vi "dos cmd test.vi"() -> ()   [LabVIEW 2010]
uses:
  <vilib>/Utility/error.llb/DialogType.ctl
panel:
  out "standard error":string
  out "standard output":string="19.0\r\n"
  in  "Numeric":dbl=9.0
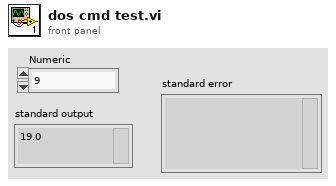
[diagram p1: front panel]
types:
  T1 = typedef "DialogType.ctl" = u16
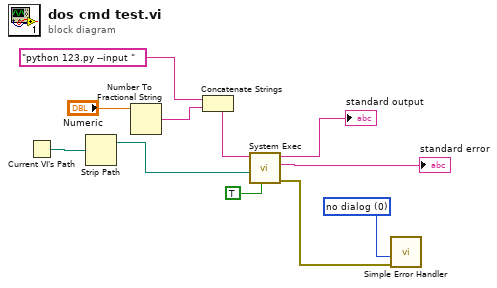
[diagram p0: block diagram]
diagram:
  w1 = T1 0 items=["no dialog", "OK message", "continue or stop message", "OK message + warnings", "continue/stop + warnings"] ("type of dialog (OK msg:1)")
  n1 = Current VI's Path() -> (path=w11:path)
  n2 = Strip Path(path=w11) -> (stripped path=w10:path)  [unwired: 1 out]
  n3 = Number To Fractional String(number="Numeric") -> (F-format string=w7:string)  [unwired: 3 in]
  n4 = Concatenate Strings("python 123.py --input ", w7) -> (w6:string)
  n5 = call <vilib>:"System Exec.vi"("run minimized? (F)"=TRUE, "working directory"=w10, "command line"=w6) -> ("error out"=w2:errorcluster, "standard error"=→"standard error":string, "standard output"=→"standard output":string)  [unwired: 5 in, 1 out]
  n6 = call <vilib>:"Simple Error Handler.vi"("type of dialog (OK msg:1)"=w1, "error in (no error)"=w2) -> ()  [unwired: 3 in, 5 out]
